vi "PartialClusters.vi"(0 "Sequence Context":T4, 2 "Cluster input":T3={"SubCluster1"={"SubCluster2"={"SubCluster3"={"SubCluster4"={"SubCluster5"={"Array OF Alumni"=[{"Name"="Andy", "Group"="A", "Classes"=["Math", "English", "Biology"]}, {"Name"="Bob", "Group"="B", "Classes"=["English", "Natural Life", "Zoology", "Numeric Analysis"]}, {"Name"="Maria", "Group"="B", "Classes"=["Spanish", "Chemistry", "Analogy of Human RelationShips", "Phisics"]}, {"Name"="Adrew", "Group"="G", "Classes"=["Math", "Calculus", "Geometry", "Computer Application"]}, {"Name"="Martha", "Group"="Q", "Classes"=["Social Behavior", "Psicology", "History of the world"]}, {"Name"="Alvin", "Group"="E", "Classes"=["Citizens of the world", "History of the Movies Industry", "TV Scripting", "Creative writing"]}], "4by4 Array"=[[[[54.0, 56.0, 56.0, 67.0, 67.0, 67.0]]], [[[0.0, 0.0, 0.0, 0.0, 0.0, 78.0]]], [[[0.0, 0.0, 0.0, 0.0, 0.0, 887.0]]], [[[0.0, 0.0, 0.0, 0.0, 0.0, 0.0]]], [[[0.0, 0.0, 0.0, 0.0, 0.0, 89.0]]], [[[0.0, 0.0, 0.0, 0.0, 0.0, 56.0]]]], "Complex Extended"=4.0+4.0i, "Complex Double"=5.0+4.0i, "Complex Single"=6.0+5.0i, "Real Matrix"=[[1.0, 2.0, 3.0], [4.0, 5.0, 6.0], [7.0, 8.0, 9.0]], "Complex Matrix"=[[1.0+0.0i, 2.0+0.0i, 3.0+0.0i], [4.0+0.0i, 5.0+0.0i, 6.0+0.0i], [7.0+0.0i, 8.0+0.0i, 9.0+0.0i]], "Waveform Chart"=0.0}}}}}}) -> (3 "Report Text":string, 4 "concatenated string":string, 5 "error out":errorcluster, 6 "x+y":cdb)   [LabVIEW 2013]
uses:
  <vilib>/addons/TestStand/_TSLegacy.llb/LabVIEW Test - Sequence Context.ctl
  <vilib>/Analysis/Matrix/Datatypes/RealMatrix.ctl
  <vilib>/Analysis/Matrix/Datatypes/ComplexMatrix.ctl
  <vilib>/Analysis/Matrix/NI_Matrix.lvlib
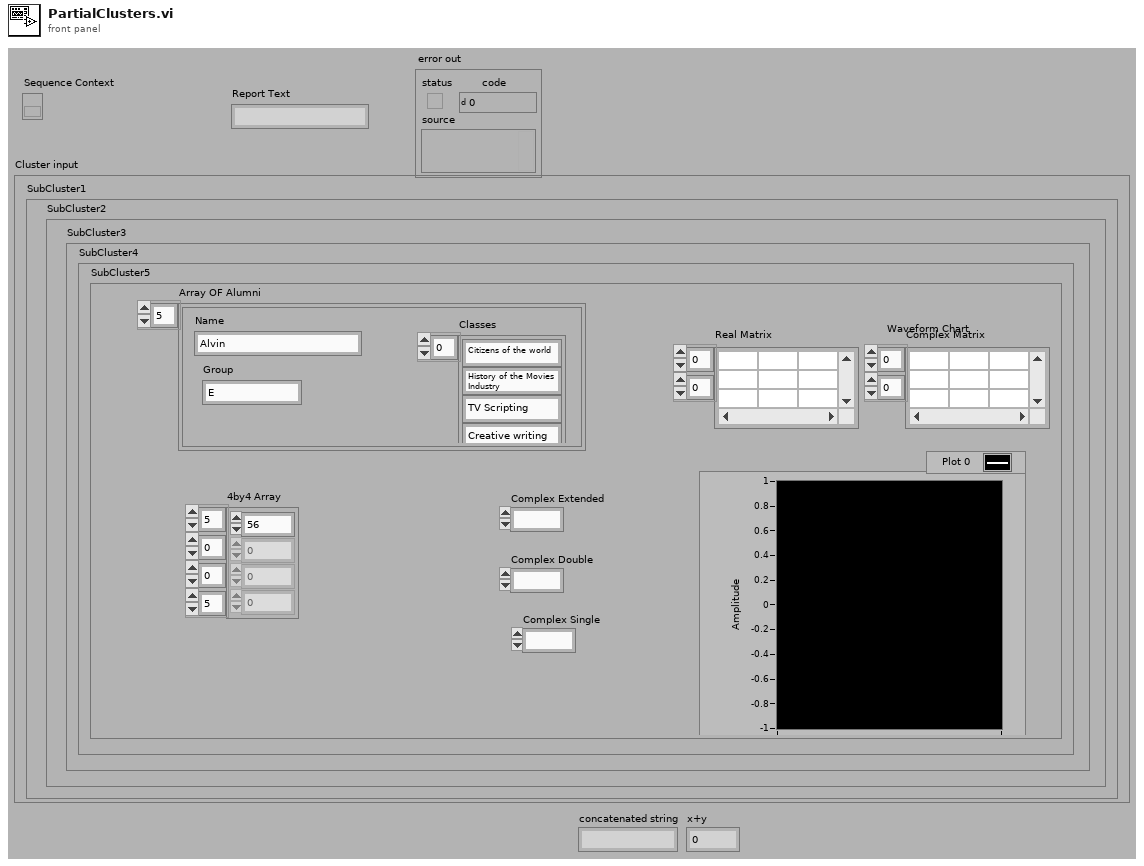
[diagram p1: front panel]
types:
  T1 = typedef "NI_Matrix.lvlib/RealMatrix.ctl" = dbl[][]
  T2 = typedef "NI_Matrix.lvlib/ComplexMatrix.ctl" = cdb[][]
  T3 = cluster{"SubCluster1":cluster{"SubCluster2":cluster{"SubCluster3":cluster{"SubCluster4":cluster{"SubCluster5":cluster{"Array OF Alumni":cluster{"Name":string, "Group":string, "Classes":string[]}[], "4by4 Array":dbl[][][][], "Complex Extended":cxt, "Complex Double":cdb, "Complex Single":csg, "Real Matrix":T1, "Complex Matrix":T2, "Waveform Chart":dbl}}}}}}
  T4 = typedef "LabVIEW Test - Sequence Context.ctl" = refnum<k7>
  T5 = cluster{"SubCluster2":cluster{"SubCluster3":cluster{"SubCluster4":cluster{"SubCluster5":cluster{"Array OF Alumni":cluster{"Name":string, "Group":string, "Classes":string[]}[], "4by4 Array":dbl[][][][], "Complex Extended":cxt, "Complex Double":cdb, "Complex Single":csg, "Real Matrix":T1, "Complex Matrix":T2, "Waveform Chart":dbl}}}}}
  T6 = cluster{"SubCluster3":cluster{"SubCluster4":cluster{"SubCluster5":cluster{"Array OF Alumni":cluster{"Name":string, "Group":string, "Classes":string[]}[], "4by4 Array":dbl[][][][], "Complex Extended":cxt, "Complex Double":cdb, "Complex Single":csg, "Real Matrix":T1, "Complex Matrix":T2, "Waveform Chart":dbl}}}}
  T7 = cluster{"SubCluster4":cluster{"SubCluster5":cluster{"Array OF Alumni":cluster{"Name":string, "Group":string, "Classes":string[]}[], "4by4 Array":dbl[][][][], "Complex Extended":cxt, "Complex Double":cdb, "Complex Single":csg, "Real Matrix":T1, "Complex Matrix":T2, "Waveform Chart":dbl}}}
  T8 = cluster{"SubCluster5":cluster{"Array OF Alumni":cluster{"Name":string, "Group":string, "Classes":string[]}[], "4by4 Array":dbl[][][][], "Complex Extended":cxt, "Complex Double":cdb, "Complex Single":csg, "Real Matrix":T1, "Complex Matrix":T2, "Waveform Chart":dbl}}
  T9 = cluster{"Array OF Alumni":cluster{"Name":string, "Group":string, "Classes":string[]}[], "4by4 Array":dbl[][][][], "Complex Extended":cxt, "Complex Double":cdb, "Complex Single":csg, "Real Matrix":T1, "Complex Matrix":T2, "Waveform Chart":dbl}
  T10 = cluster{"Name":string, "Group":string, "Classes":string[]}[]
  T11 = cluster{"Name":string, "Group":string, "Classes":string[]}
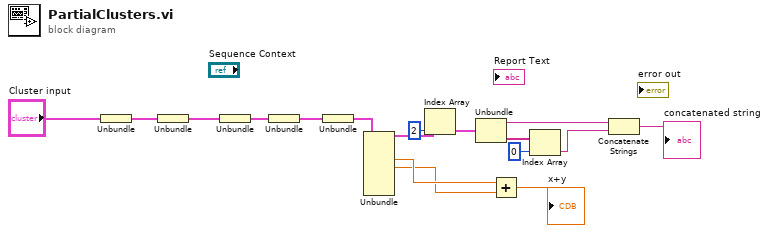
[diagram p0: block diagram]
diagram:
  n1 = Unbundle("Cluster input") -> ("SubCluster1"=w16:T5)
  n2 = Unbundle(w16) -> ("SubCluster2"=w15:T6)
  n3 = Unbundle(w15) -> ("SubCluster3"=w14:T7)
  n4 = Unbundle(w14) -> ("SubCluster4"=w13:T8)
  n5 = Unbundle(w13) -> ("SubCluster5"=w12:T9)
  n6 = Unbundle(w12) -> ("Array OF Alumni"=w11:T10, "Complex Double"=w3:cdb, "Complex Single"=w2:csg)  [unwired: 5 out]
  n7 = Index Array(array=w11, index=2) -> (element=w9:T11)
  n8 = Unbundle(w9) -> ("Name"=w6:string, "Classes"=w8:string[])  [unwired: 1 out]
  n9 = Add(x=w3, y=w2) -> (x+y=→"x+y":cdb)
  n10 = Index Array(array=w8, index=0) -> (element=w5:string)
  n11 = Concatenate Strings(w6, w5) -> (→"concatenated string":string)
